vi "FGV_Timer_ex_4.vi"(7 "Timer action (run)":T1=enum."Run", 8 "error in (no error)":errorcluster) -> (0 "error out":errorcluster, 3 "Time Elapsed":dbl)   [LabVIEW 2020]
uses:
  #typedef_FGV_TimerAction_ex_4.ctl
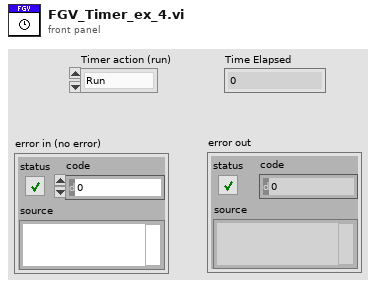
[diagram p1: front panel]
types:
  T1 = typedef "#typedef_FGV_TimerAction_ex_4.ctl" = enum16{"Reset", "Run", "Pause"}
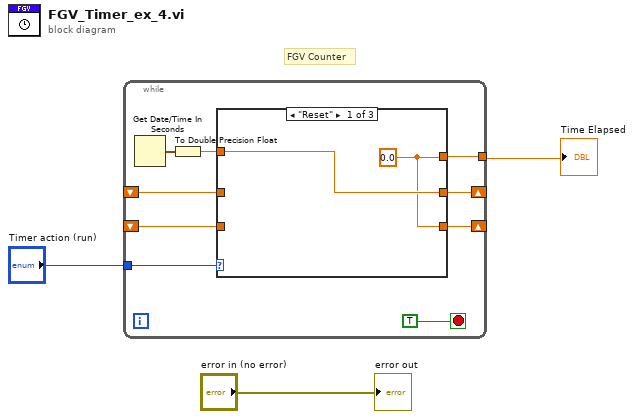
[diagram p0: block diagram]
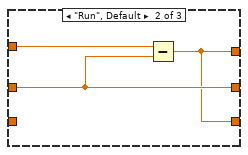
[diagram p2: hidden frame]
diagram:
  # "FGV Counter"
  n1 = while {
    tunnel: "Timer action (run)" -> [w12]
    shift-right: [w9] -> _
    shift-left: _ -> [w7]
    tunnel: [w6] -> w3
    shift-right: [w5] -> _
    shift-left: _ -> [w4]
    stop <- TRUE stop-if-true
    n2 = Get Date/Time In Seconds() -> (seconds since 1Jan1904=w10:timestamp)
    n3 = To Double Precision Float(number=w10) -> (double precision float=w8:dbl)
    n4 = case shown="\"Reset\"" w12 {
      tunnel: [w14 w16 w19] -> w9
      tunnel: w8 -> [w14 w17 _]
      tunnel: w7 -> [_ w16 w19]
      tunnel: [w13 w15 w18] -> w6
      tunnel: [w13 w15 w18] -> w5
      tunnel: w4 -> [_ _ w18]
      frame "Reset" {
        w13 = 0.0
      }
      frame "Run", Default {
        n5 = Subtract(x=w17, y=w16) -> (x-y=w15:dbl)
      }
      frame "Pause" {
      }
    }
  }
  "Time Elapsed" <- w3
  "error out" <- "error in (no error)"
